vi "Read Path Too Long To Fit.vi"(9 "Path in":refnum<class "Path.lvclass">) -> (3 "Path out":refnum<class "Path.lvclass">, 4 "Path Too Long To Fit":enum32{"Abbreviate Path", "Clip Path"}(ring))   [LabVIEW 2014, in "Path.lvclass"]
uses:
  Path.lvclass
  Path.lvclass/Path.ctl
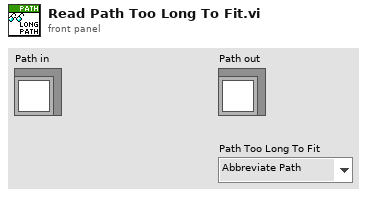
[diagram p1: front panel]
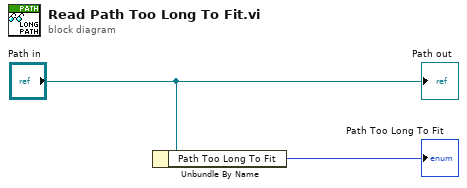
[diagram p0: block diagram]
diagram:
  n1 = Unbundle By Name("Path in") -> ("Path Too Long To Fit"=→"Path Too Long To Fit":enum32{"Abbreviate Path", "Clip Path"})
  "Path out" <- "Path in"
